vi "Boron Rod.vi"() -> ()   [LabVIEW 2020]
uses:
  <vilib>/Utility/miscctls.llb/LVAnnotationListTypeDef.ctl
  070368b1-a1f6-40e9-b446-795936455d25.vi
  <vilib>/Analysis/3filter.llb/Savitzky-Golay Filter (DBL).vi
  global/SettingVariable.vi
  <vilib>/Analysis/NI_AAL_SigProc.lvlib
  <vilib>/Analysis/NI_AALPro.lvlib
  <vilib>/Analysis/NI_AALBase.lvlib
panel:
  out "历史波形图":cluster{dbl, dbl, dbl[][]}(graph)
  in  "width":i32=60
  in  "选择反应性：":enum16{""}(ring)
  out "左选标时刻":timestamp caption="左选标时刻：" format="%<%.2X %x>T"
  out "数据点数":i32 caption="选中的数据点数："
  in  "拟合直线":bool
  out "采样间隔":dbl
  out "开始时间":timestamp
  in  "在线数据":bool
  in  "打开文件":bool
  out "反应性记录表":string[][](table) caption="计算结果记录表"
  in  "保存表格":bool
  in  "添加记录":bool
  out "提示信息":string="打开文件后，拖动波形图中的游标选取数据进行计算。"
  out "文件信息":string
  # "坐标轴与图例"
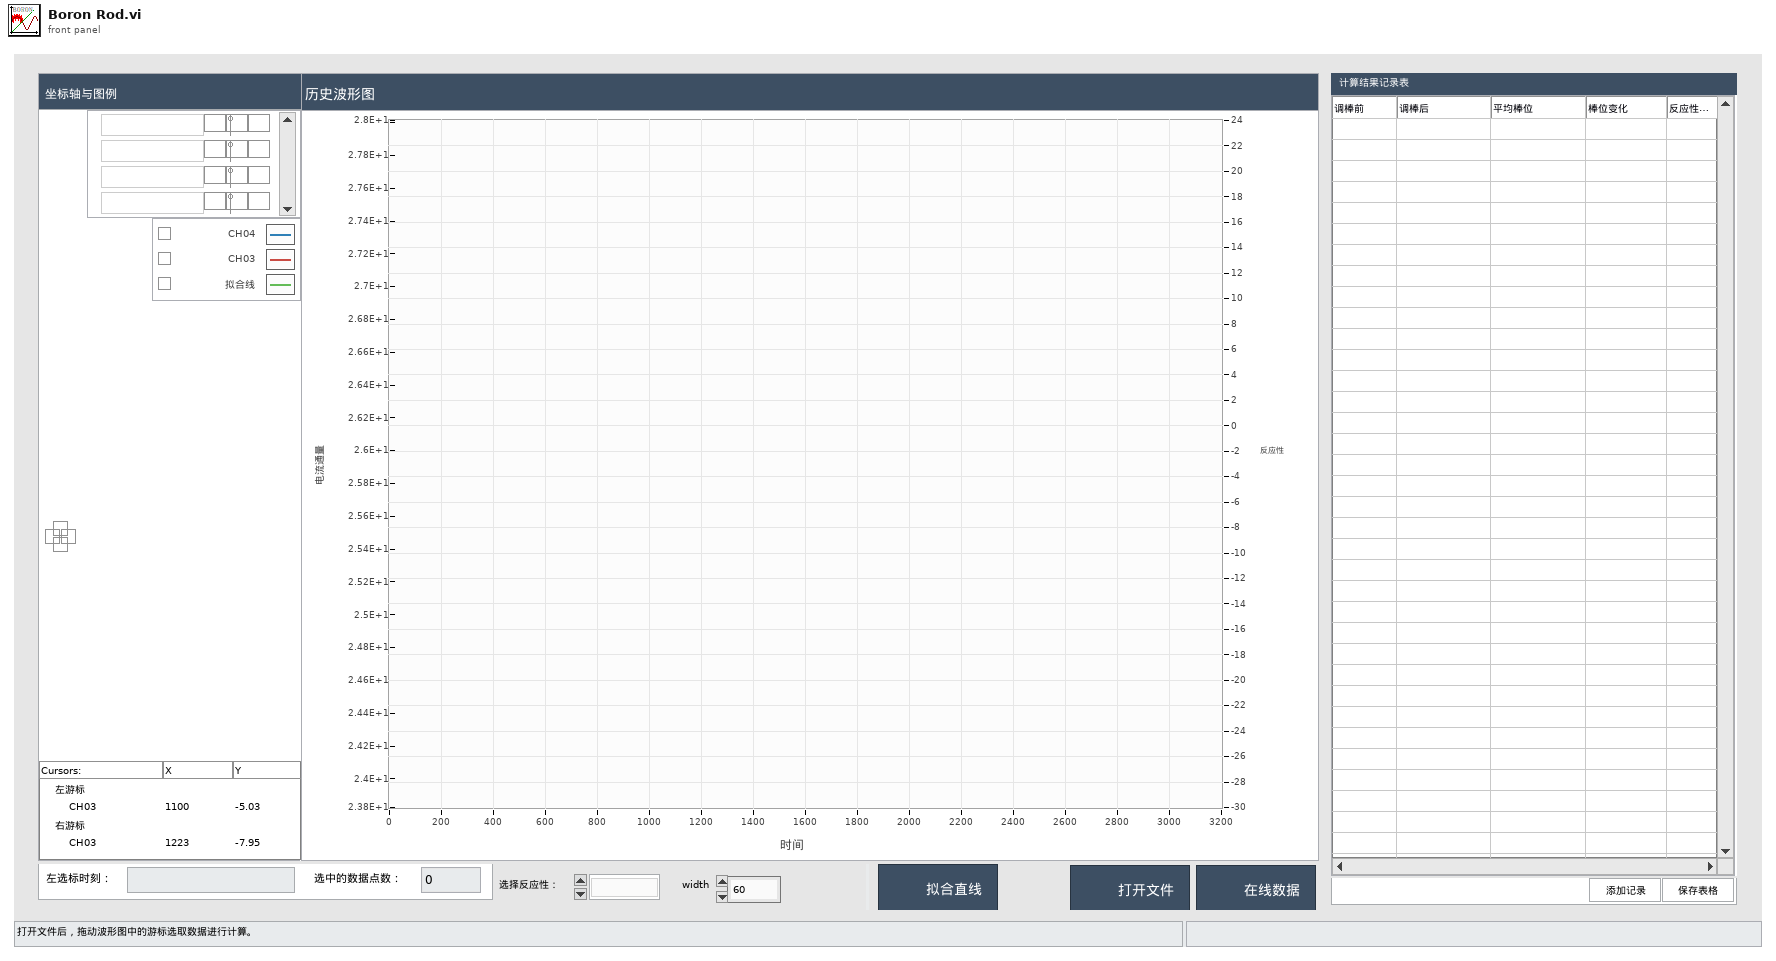
[diagram p1: front panel]
types:
  T1 = typedef "LVAnnotationListTypeDef.ctl" = cluster{"Name":string, "Color":u32, "Style":u8, "Point Style":u8, "Name Visible":bool, "Allow Drag":bool, "Annotation Mode":u32, "Plot":i32, "Index":i32, "Position":cluster{"X":dbl, "Y":dbl}, "X Scale":u32, "Y Scale":u32, "Show Arrow":bool, "Lock Name":bool, "Plot Area":i32, "Label Offset":cluster{"X":dbl, "Y":dbl}}[]
  T2 = cluster{"Name":string, "Color":u32, "Style":u8, "Point Style":u8, "Name Visible":bool, "Allow Drag":bool, "Annotation Mode":u32, "Plot":i32, "Index":i32, "Position":cluster{"X":dbl, "Y":dbl}, "X Scale":u32, "Y Scale":u32, "Show Arrow":bool, "Lock Name":bool, "Plot Area":i32, "Label Offset":cluster{"X":dbl, "Y":dbl}}
  T3 = enum16{"open", "replace", "create", "open or create", "replace or create", "replace or create with confirmation"}
  T4 = typedef "LVCursorListTypeDef.ctl" = cluster{"Name":string, "Color":u32, "Style":u8, "Point Style":u8, "Name Visible":bool, "Allow Drag":bool, "Cursor Mode":u32, "Plot":i32, "Index":i32, "Position":cluster{"X":dbl, "Y":dbl}, "X Scale":u32, "Y Scale":u32, "Watch Plots":i32[], "Watch All Plots":bool, "Plot Area":i32, "Label Offset":cluster{"X":dbl, "Y":dbl}}[]
  T5 = cluster{"Name":string, "Color":u32, "Style":u8, "Point Style":u8, "Name Visible":bool, "Allow Drag":bool, "Cursor Mode":u32, "Plot":i32, "Index":i32, "Position":cluster{"X":dbl, "Y":dbl}, "X Scale":u32, "Y Scale":u32, "Watch Plots":i32[], "Watch All Plots":bool, "Plot Area":i32, "Label Offset":cluster{"X":dbl, "Y":dbl}}
  T6 = enum32{"invalid app kind", "Development System", "Run Time System", "Student Edition", "Embedded LabVIEW", "Evaluation", "Custom"}
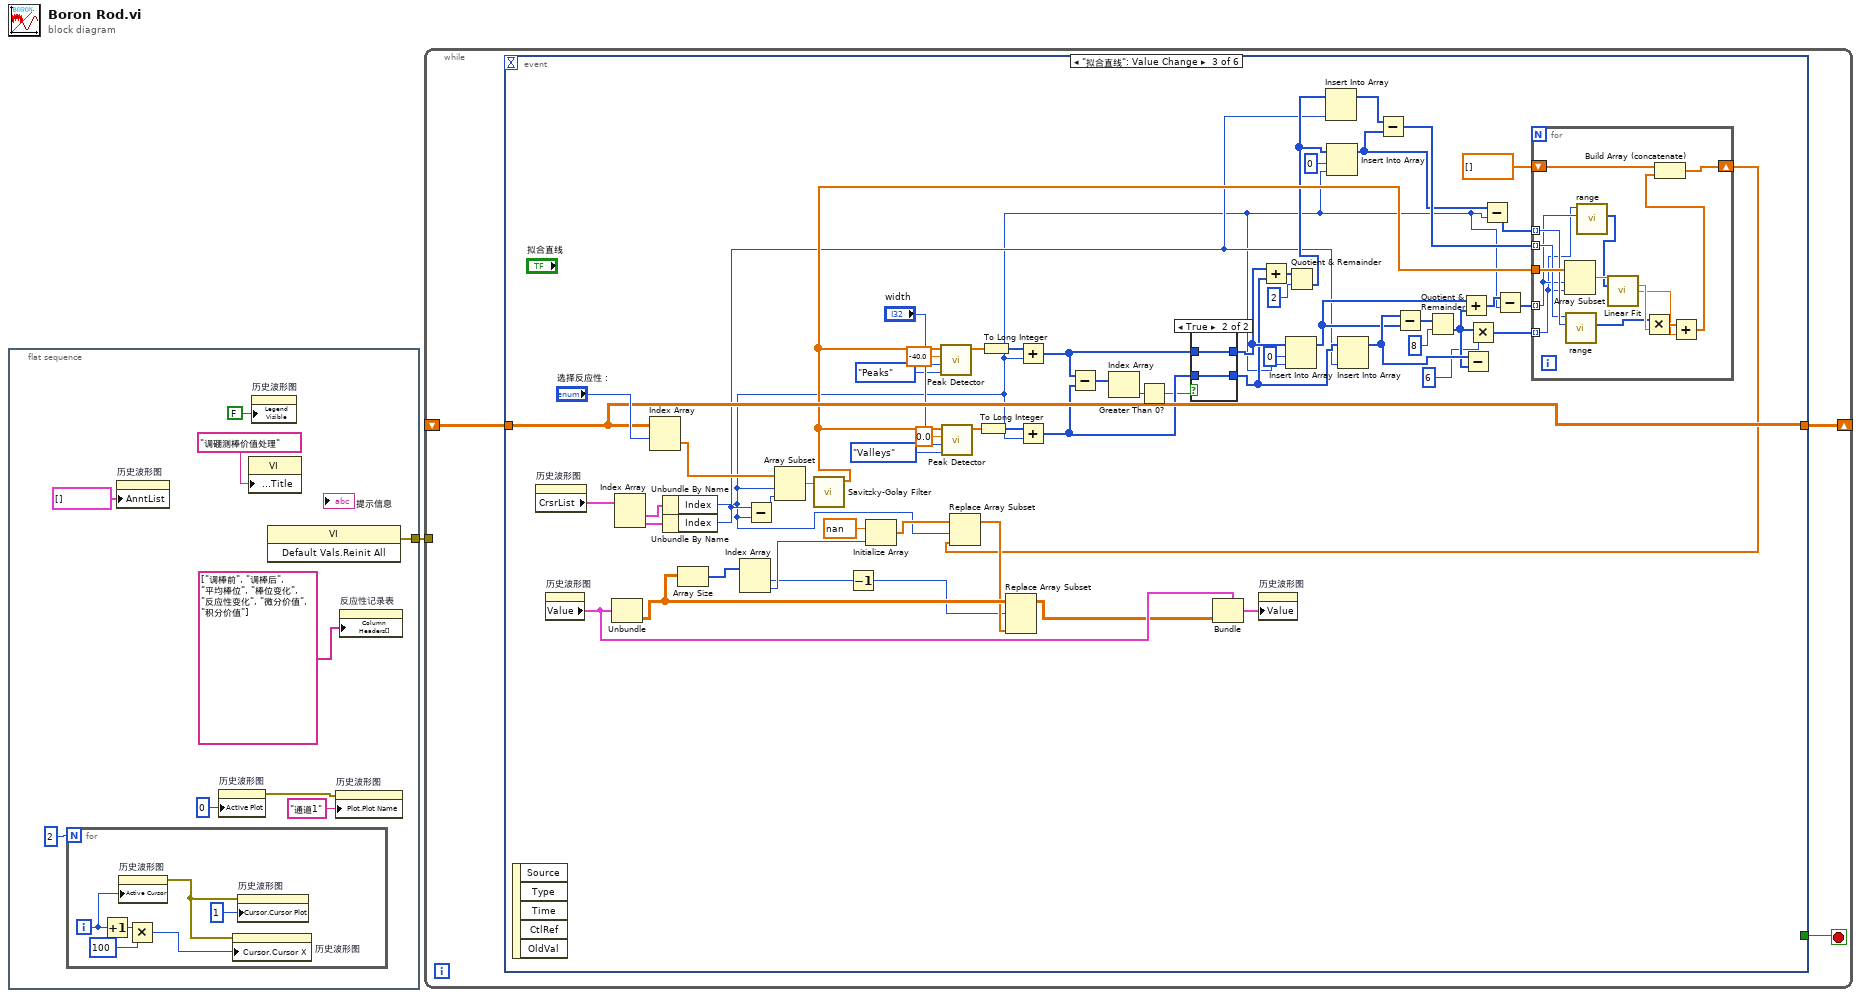
[diagram p0: block diagram]
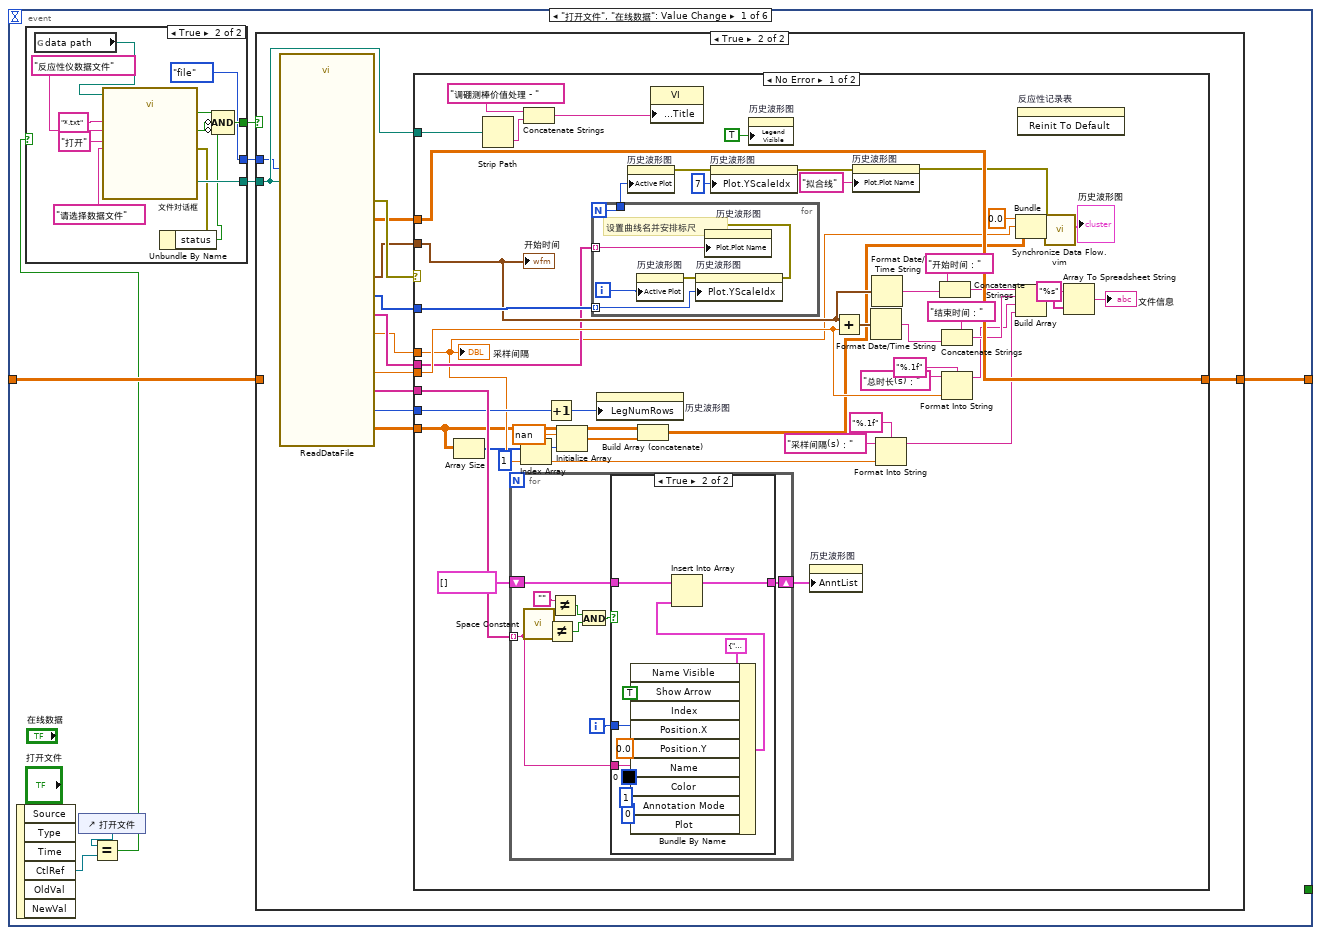
[diagram p2: hidden frame]
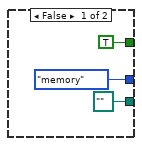
[diagram p3: hidden frame]
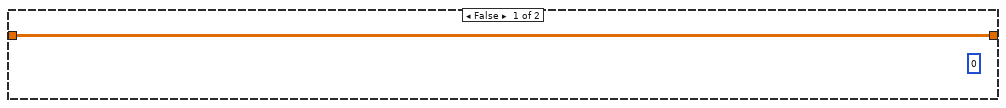
[diagram p4: hidden frame]
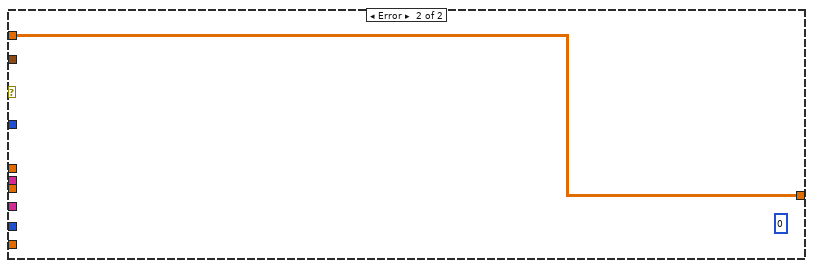
[diagram p6: hidden frame]
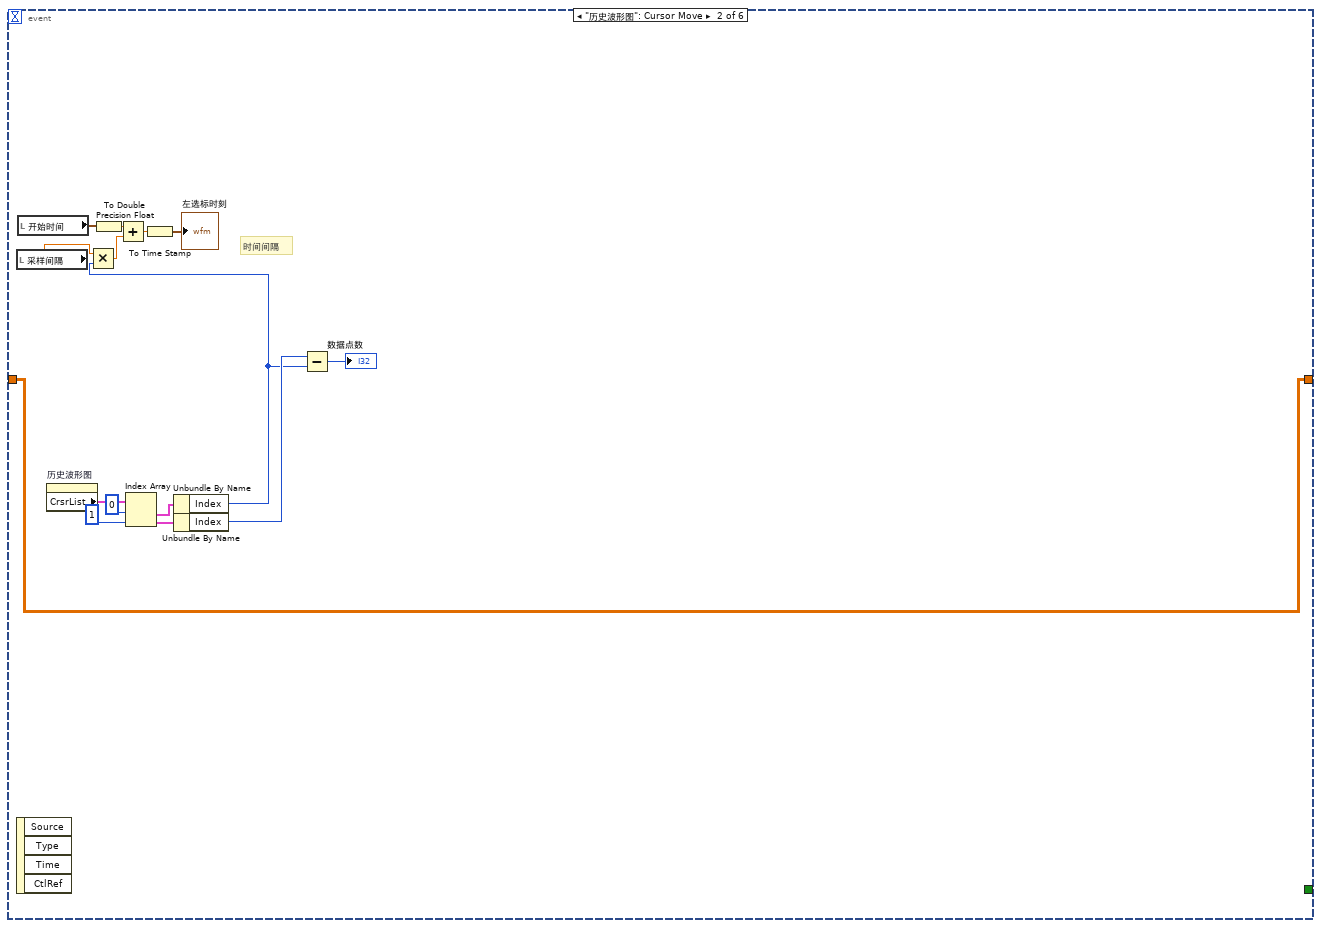
[diagram p7: hidden frame]
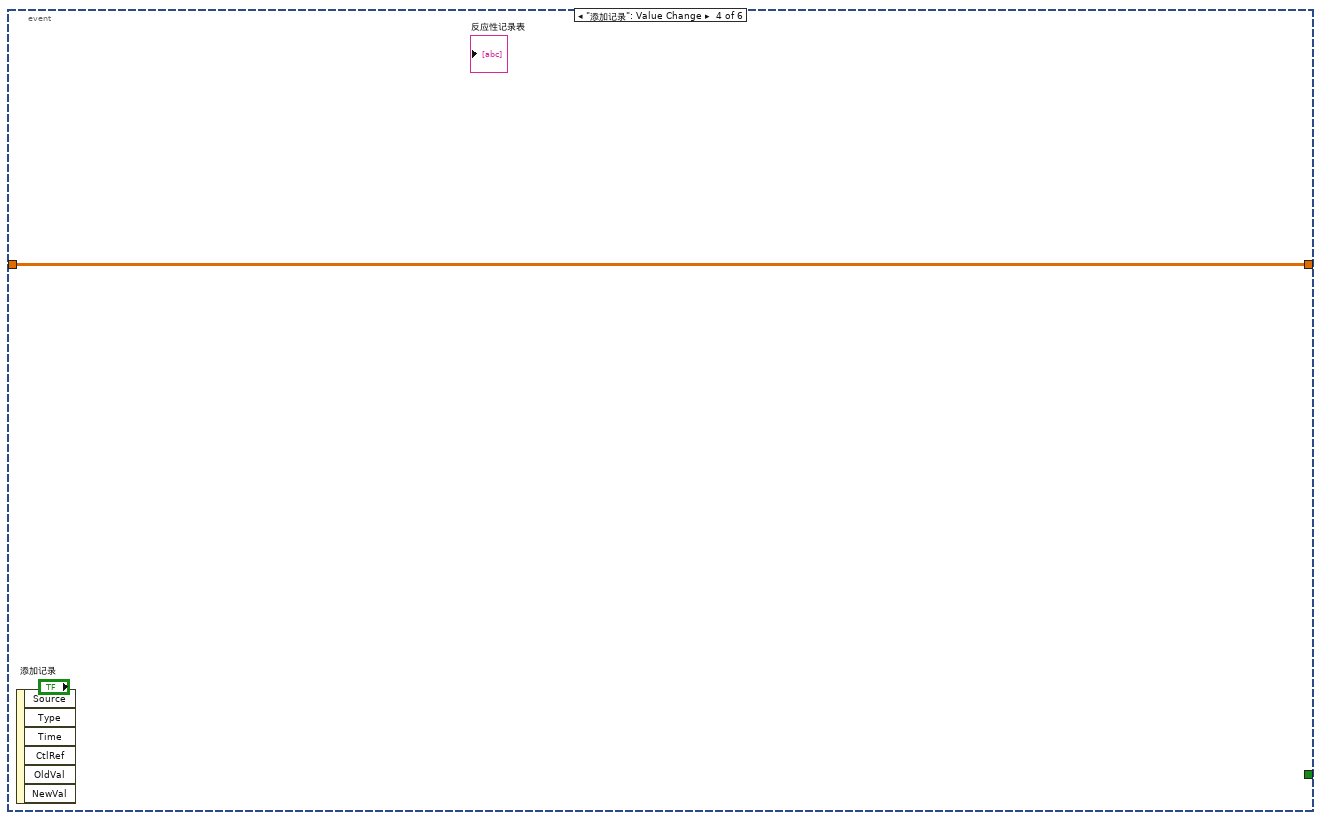
[diagram p9: hidden frame]
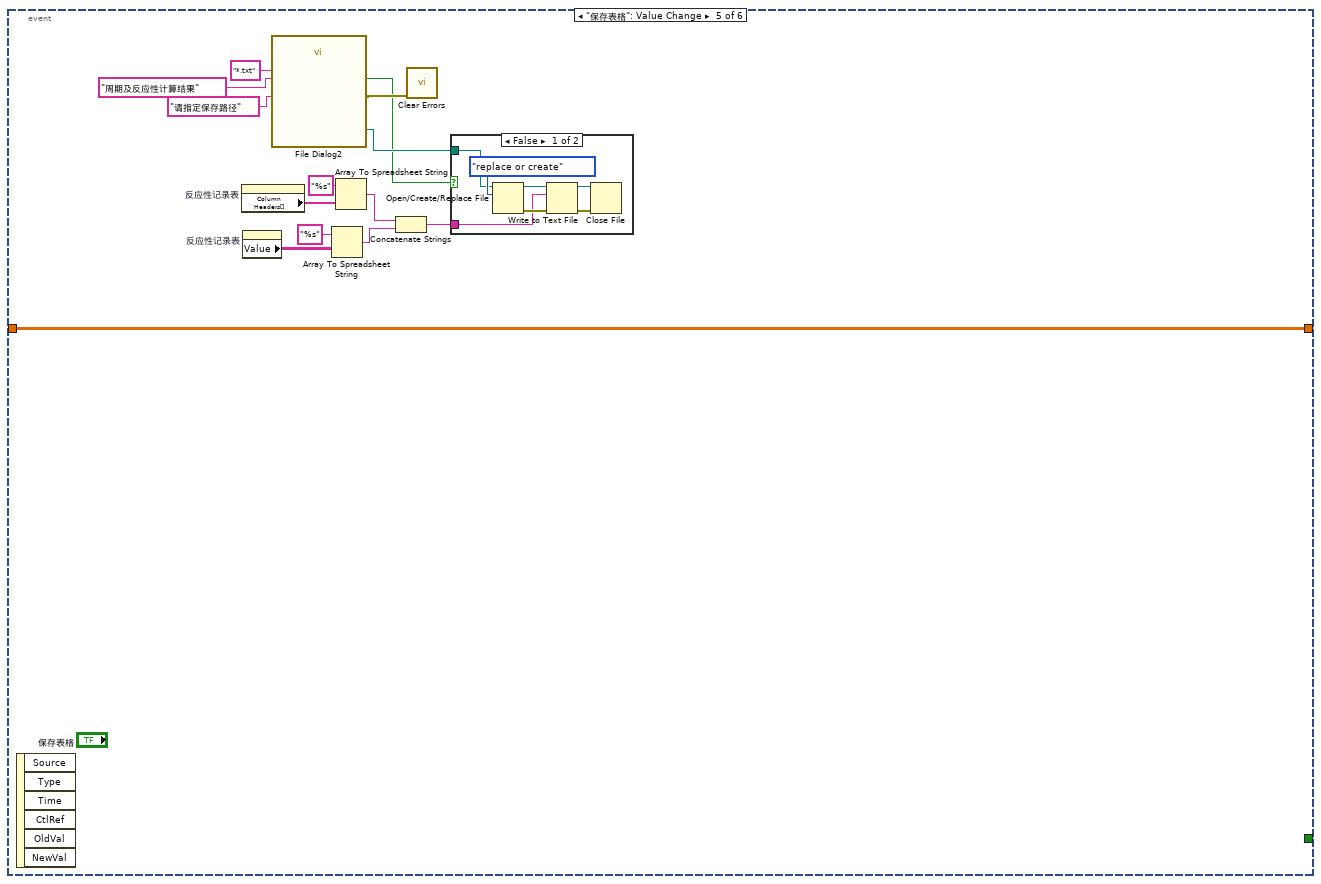
[diagram p10: hidden frame]
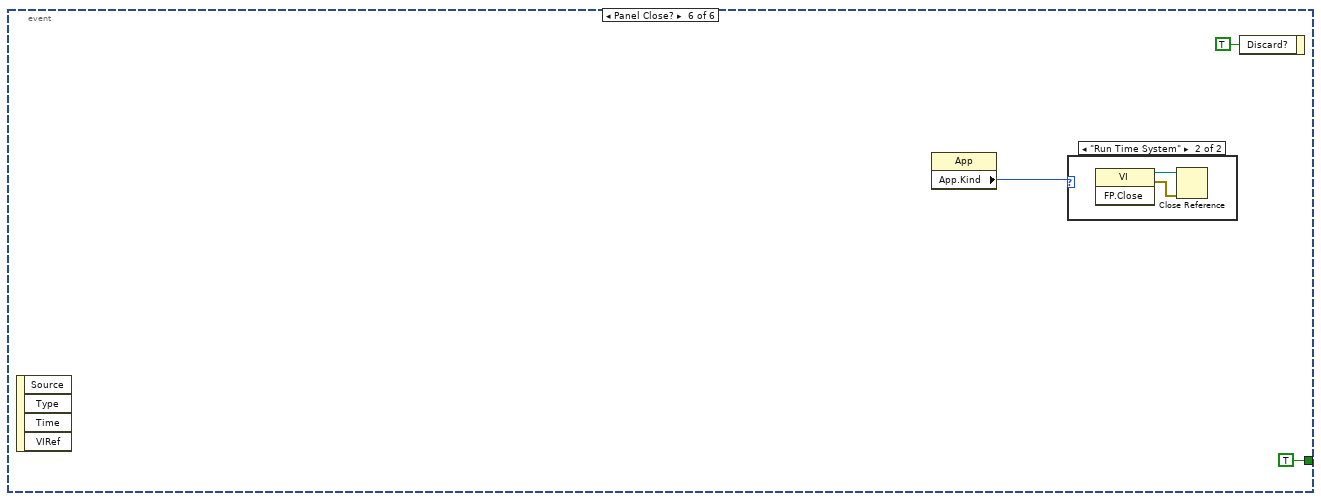
[diagram p12: hidden frame]
diagram:
  n1 = flat-sequence {
    tunnel: [w6] -> w1
    frame #0 {
      n2 = for {
        N: 2 -> [_]
        i -> [w15]
        n3 = Increment(x=w15) -> (x+1=w14:i32)
        n4 = property on="历史波形图" class="WFGraph (strict)"("Active Cursor"=w15) -> (error out=w11:errorcluster)  [unwired: 2 in, 1 out]
        n5 = Multiply(x=w14, y=100) -> (x*y=w12:i32)
        n6 = property on="历史波形图" class="WFGraph (strict)"(error in=w11, "Cursor.Cursor X"=w12) -> ()  [unwired: 1 in, 2 out]
        n7 = property on="历史波形图" class="WFGraph (strict)"(error in=w11, "Cursor.Cursor Plot"=1 ("Cursor.Cursor Index")) -> ()  [unwired: 1 in, 2 out]
      }
      n8 = property on="历史波形图" class="WFGraph (strict)"("AnntList"=T1 [] ("Annotation List")) -> ()  [unwired: 2 in, 2 out]
      n9 = property on="历史波形图" class="WFGraph (strict)"("Active Plot"=u32 0) -> (error out=w8:errorcluster)  [unwired: 2 in, 1 out]
      n10 = property class="VI"("Front Panel.Title"="调硼测棒价值处理" ("Front Panel Window:Title")) -> ()  [unwired: 2 in, 2 out]
      n11 = property on="历史波形图" class="WFGraph (strict)"("Legend Visible"=FALSE ("Legend:Visible")) -> ()  [unwired: 2 in, 2 out]
      n12 = invoke class="VI" method="Default Vals.Reinit All"() -> (error out=w6:errorcluster)  [unwired: 3 in, 2 out]
      n13 = property on="历史波形图" class="WFGraph (strict)"(error in=w8, "Plot.Plot Name"="通道1") -> ()  [unwired: 1 in, 2 out]
      n14 = property on="反应性记录表" class="Tbl (strict)"("Column Headers[]"=string[] ["调棒前", "调棒后", "平均棒位", "棒位变化", "反应性变化", "微分价值", "积分价值"] ("行首字符串[]")) -> ()  [unwired: 2 in, 2 out]
    }
  }
  n15 = while {
    shift-right: [w19] -> _
    shift-left: _ -> [w18]
    tunnel: w1 -> [_]
    stop <- w17 stop-if-true
    n16 = event shown="[2] \"拟合直线\": Value Change" {
      selector: _ -> [_ _ _ _ _ _]
      dyn-events: _ -> [_ _ _ _ _ _]
      timeout: _ -> [_ _ _ _ _ _]
      tunnel: [w26 w137 w190 w224 w238 _] -> w19
      tunnel: w18 -> [w25 w137 w190 w224 w238 _]
      tunnel: [_ _ _ _ _ TRUE] -> w17
      event "打开文件", "在线数据": Value Change {
        n17 = event-data() -> ("CtlRef"=w23:refnum<vi>)  [unwired: 1 in, 5 out]
        n18 = control-ref of="打开文件"() -> (w22:refnum<vi>)
        n19 = Equal?(x=w22, y=w23) -> (x = y?=w21:bool)
        n20 = case shown="True" w21 {
          tunnel: [path "" ("selected path") w42] -> w27
          tunnel: [TRUE w33] -> w24
          tunnel: [enum16{"file", "memory"}."memory" ("source") enum16{"file", "memory"}."file" ("source")] -> w20
          frame False {
          }
          frame True {
            n21 = global read "SettingVariable.vi" "data path"() -> (w32:path)
            n22 = call "文件对话框"("start path"=w32, "prompt"="请选择数据文件", "button label"="打开", "pattern (all files)"="*.txt", "pattern label"="反应性仪数据文件") -> ("selected path"=w42:path, "exists"=w36:bool, "cancelled"=w35:bool, "error out"=w37:errorcluster)  [unwired: 7 in]
            n23 = Unbundle By Name(w37) -> ("status"=w34:bool)
            n24 = Compound Arithmetic op=AND(w36, invert w35, invert w34) -> (w33:bool)
          }
        }
        n25 = case shown="True" w24 {
          tunnel: w27 -> [_ w46]
          tunnel: [w43 w48] -> w26
          tunnel: w25 -> [w43 _]
          tunnel: w20 -> [_ w45]
          frame False {
            (unwired) 0 ("曲线数")
          }
          frame True {
            n26 = call "ReadDataFile.vi"("file path"=w46, "source"=w45) -> ("曲线对应标尺编号"=w52:i32[], "全部数据"=w44:dbl[][], "曲线名"=w51:string[], "时间间隔"=w50:dbl, "曲线数"=w54:i32, "开始时间"=w47:timestamp, "反应性数据"=w49:dbl[][], "总时长(s)"=w55:dbl, "error out"=w56:errorcluster, "备注数组"=w53:string[])  [unwired: 1 in, 3 out]
            n27 = case shown="No Error" w56 {
              tunnel: w55 -> [w93 _]
              tunnel: w54 -> [w75 _]
              tunnel: w53 -> [w102 _]
              tunnel: w52 -> [w101 _]
              tunnel: w51 -> [w81 _]
              tunnel: w50 -> [w67 _]
              tunnel: w49 -> [w100 w132]
              tunnel: [w100 w132] -> w48
              tunnel: w47 -> [w98 _]
              tunnel: w46 -> [w77 _]
              tunnel: w44 -> [w63 _]
              frame No Error {
                n28 = Array Size(array=w63) -> (size(s)=w65:i32[])
                n29 = Strip Path(path=w77) -> (name=w78:string)  [unwired: 1 out]
                n30 = for {
                  tunnel: w102 -> [w114] mode=indexing
                  shift-right: [w116] -> w104
                  shift-left: T1 [] ("注释列表") -> [w117]
                  i -> [w118]
                  n31 = call <vilib>:"Space Constant.vi"() -> ("String"=w119:string)
                  n32 = Not Equal?(x=w119, y=w114) -> (x != y?=w112:bool)
                  n33 = Not Equal?(x="", y=w114) -> (x != y?=w113:bool)
                  n34 = And(x=w113, y=w112) -> (x .and. y?=w111:bool)
                  n35 = case shown="True" w111 {
                    tunnel: w114 -> [_ w126]
                    tunnel: w118 -> [_ w128]
                    tunnel: w117 -> [w120 w131]
                    tunnel: [w120 w130] -> w116
                    frame False {
                    }
                    frame True {
                      w129 = TRUE ("Show Arrow")
                      n36 = Bundle By Name(cluster=T2 {"Name"="", "Color"=0, "Style"=0, "Point Style"=0, "Name Visible"=FALSE, "Allow Drag"=FALSE, "Annotation Mode"=0, "Plot"=0, "Index"=0, "Position"={"X"=0.0, "Y"=0.0}, "X Scale"=0, "Y Scale"=0, "Show Arrow"=FALSE, "Lock Name"=FALSE, "Plot Area"=0, "Label Offset"={"X"=0.0, "Y"=0.0}} ("元素"), "Name Visible"=w129, "Show Arrow"=w129, "Index"=w128, "Position.X"=w128, "Position.Y"=0.0 ("Y"), "Name"=w126, "Color"=u32 0, "Annotation Mode"=u32 1, "Plot"=0) -> (w127:T2)
                      n37 = Insert Into Array(array=w131, new element=w127) -> (w130:T1)  [unwired: 1 in]
                    }
                  }
                }
                n38 = Index Array(array=w65, index=1) -> (element=w62:i32)
                n39 = Concatenate Strings("调硼测棒价值处理 - " ("string"), w78) -> (w79:string)
                n40 = Increment(x=w75) -> (x+1=w57:i32)
                n41 = Initialize Array(nan, w62) -> (w60:dbl[])
                n42 = for {
                  N -> [w105]
                  tunnel: w101 -> [w108] mode=indexing
                  tunnel: w81 -> [w106] mode=indexing
                  tunnel: [w105] -> w70
                  i -> [w107]
                  # "设置曲线名并安排标尺"
                  n43 = property on="历史波形图" class="WFGraph (strict)"("Active Plot"=w107) -> (error out=w110:errorcluster)  [unwired: 2 in, 1 out]
                  n44 = property on="历史波形图" class="WFGraph (strict)"(error in=w110, "Plot.YScaleIdx"=w108) -> (error out=w109:errorcluster)  [unwired: 1 in, 1 out]
                  n45 = property on="历史波形图" class="WFGraph (strict)"(error in=w109, "Plot.Plot Name"=w106) -> ()  [unwired: 1 in, 2 out]
                }
                n46 = property on="历史波形图" class="WFGraph (strict)"("LegNumRows"=w57) -> ()  [unwired: 2 in, 2 out]
                n47 = property on="历史波形图" class="WFGraph (strict)"("Active Plot"=w70) -> (error out=w72:errorcluster)  [unwired: 2 in, 1 out]
                n48 = Build Array (concatenate)(w63, w60) -> (w66:dbl[][])
                n49 = property class="VI"("Front Panel.Title"=w79) -> ()  [unwired: 2 in, 2 out]
                n50 = property on="历史波形图" class="WFGraph (strict)"(error in=w72, "Plot.YScaleIdx"=u32 7 ("Plot.Y Scale Index")) -> (error out=w73:errorcluster)  [unwired: 1 in, 1 out]
                n51 = property on="历史波形图" class="WFGraph (strict)"("Legend Visible"=TRUE ("Legend:Visible")) -> ()  [unwired: 2 in, 2 out]
                n52 = property on="历史波形图" class="WFGraph (strict)"("AnntList"=w104) -> ()  [unwired: 2 in, 2 out]
                n53 = Add(x=w98, y=w93) -> (x+y=w99:timestamp)
                n54 = property on="历史波形图" class="WFGraph (strict)"(error in=w73, "Plot.Plot Name"="拟合线") -> (error out=w58:errorcluster)  [unwired: 1 in, 1 out]
                n55 = Format Date/Time String(seconds (now)=w99) -> (date/time string=w94:string)  [unwired: 2 in]
                n56 = Format Date/Time String(seconds (now)=w98) -> (date/time string=w96:string)  [unwired: 2 in]
                n57 = Format Into String(format string="%.1f", initial string="采样间隔(s)：", w67) -> (resulting string=w85:string)  [unwired: 1 in, 1 out]
                n58 = Concatenate Strings("开始时间：" ("string"), w96) -> (w90:string)
                n59 = Concatenate Strings("结束时间：" ("string"), w94) -> (w87:string)
                n60 = Format Into String(format string="%.1f", initial string="总时长(s)：", w93) -> (resulting string=w86:string)  [unwired: 1 in, 1 out]
                n61 = Bundle(0.0, "时间间隔"=w67, w66) -> (w69:cluster{dbl, "时间间隔":dbl, dbl[][]})  [unwired: 1 in]
                n62 = Build Array(w90, w87, w86, w85) -> (w89:string[])
                n63 = invoke on="反应性记录表" class="Tbl (strict)" method="Reinit To Default"() -> ()  [unwired: 3 in, 3 out]
                n64 = call "Synchronize Data Flow.vim"("input 2"=w69, "input 1"=w58) -> ("output 2"=→"历史波形图":cluster{dbl, "时间间隔":dbl, dbl[][]})  [unwired: 2 in, 3 out]
                n65 = Array To Spreadsheet String(array=w89, 3:"%s" ("format string")) -> (spreadsheet string=→"文件信息":string)  [unwired: 1 in]
                "开始时间" <- w98
                "采样间隔" <- w67
              }
              frame Error {
                (unwired) 0 ("曲线数")
              }
            }
          }
        }
      }
      event "历史波形图": Cursor Move {
        # "时间间隔"
        n66 = local read "采样间隔"() -> (w135:dbl)
        n67 = event-data() -> ()  [unwired: 1 in, 4 out]
        n68 = local read "开始时间"() -> (w136:timestamp)
        n69 = property on="历史波形图" class="WFGraph (strict)"() -> ("CrsrList"=w143:T4)  [unwired: 2 in, 2 out]
        n70 = To Double Precision Float(number=w136) -> (double precision float=w142:dbl)
        n71 = Index Array(array=w143, index #1=0 ("index"), index #2=1 ("index")) -> (element #1=w145:T5, element #2=w147:T5)
        n72 = Unbundle By Name(w145) -> ("Index"=w133:i32)
        n73 = Multiply(x=w135, y=w133) -> (x*y=w139:dbl)
        n74 = Add(x=w142, y=w139) -> (x+y=w141:dbl)
        n75 = To Time Stamp(1:w141) -> (0:→"左选标时刻":timestamp)
        n76 = Unbundle By Name(w147) -> ("Index"=w138:i32)
        n77 = Subtract(x=w138, y=w133) -> (x-y=→"数据点数":i32)
      }
      event "拟合直线": Value Change {
        n78 = event-data() -> ()  [unwired: 1 in, 5 out]
        n79 = property on="历史波形图" class="WFGraph (strict)"() -> ("CrsrList"=w203:T4)  [unwired: 2 in, 2 out]
        n80 = property on="历史波形图" class="WFGraph (strict)"() -> ("Value"=w193:cluster{dbl, dbl, dbl[][]})  [unwired: 2 in, 2 out]
        n81 = Unbundle(w193) -> (w199:dbl[][])  [unwired: 2 out]
        n82 = Index Array(array=w203) -> (element #1=w204:T5, element #2=w205:T5)  [unwired: 2 in]
        n83 = Index Array(array=w190, index (row)="选择反应性：") -> (element=w201:dbl[])  [unwired: 1 in]
        n84 = Unbundle By Name(w204) -> ("Index"=w149:i32)
        n85 = Unbundle By Name(w205) -> ("Index"=w155:i32)
        n86 = Array Size(array=w199) -> (size(s)=w198:i32[])
        n87 = Index Array(array=w198) -> (element #1=w194:i32, element #2=w197:i32)  [unwired: 2 in]
        n88 = Subtract(x=w155, y=w149) -> (x-y=w200:i32)
        n89 = Array Subset(array=w201, index=w149, length=w200) -> (w163:dbl[])
        n90 = call-poly <vilib>:"Savitzky-Golay Filter.vi"("X"=w163) -> ("Filtered X"=w162:dbl[])  [unwired: 9 in, 1 out]
        n91 = Decrement(x=w194) -> (x-1=w189:i32)
        n92 = Initialize Array(nan ("element"), w197) -> (w188:dbl[])
        n93 = call <vilib>:"Peak Detector.vi"("peaks/valleys"=enum32{"Peaks", "Valleys"}."Peaks", "width"="width", "threshold"=-40.0, "X"=w162) -> ("Locations"=w187:dbl[])  [unwired: 3 in, 4 out]
        n94 = call <vilib>:"Peak Detector.vi"("peaks/valleys"=enum32{"Peaks", "Valleys"}."Valleys", "width"="width", "threshold"=0.0, "X"=w162) -> ("Locations"=w183:dbl[])  [unwired: 3 in, 4 out]
        n95 = To Long Integer(number=w183) -> (32bit integer=w179:i32[])
        n96 = To Long Integer(number=w187) -> (32bit integer=w180:i32[])
        n97 = Add(x=w180, y=w149) -> (x+y=w168:i32[])
        n98 = Add(x=w179, y=w149) -> (x+y=w167:i32[])
        n99 = Subtract(x=w168, y=w167) -> (x-y=w181:i32[])
        n100 = Index Array(array=w181) -> (element=w182:i32)  [unwired: 1 in]
        n101 = Greater Than 0?(x=w182) -> (x > 0?=w166:bool)
        n102 = case shown="True" w166 {
          tunnel: [w206 w209] -> w161
          tunnel: w168 -> [w207 w209]
          tunnel: [w207 w208] -> w160
          tunnel: w167 -> [w206 w208]
          frame False {
          }
          frame True {
          }
        }
        n103 = Add(x=w161, y=w160) -> (x+y=w159:i32[])
        n104 = Insert Into Array(array=w161, index=0, new element=w149) -> (w172:i32[])
        n105 = Quotient & Remainder(x=w159, y=2) -> (floor(x/y)=w156:i32[])  [unwired: 1 out]
        n106 = Insert Into Array(array=w156, new element=w155) -> (w154:i32[])  [unwired: 1 in]
        n107 = Insert Into Array(array=w156, index=0, new element=w149) -> (w151:i32[])
        n108 = Insert Into Array(array=w160, new element=w155) -> (w176:i32[])  [unwired: 1 in]
        n109 = Subtract(x=w154, y=w151) -> (x-y=w153:i32[])
        n110 = Subtract(x=w176, y=w172) -> (x-y=w171:i32[])
        n111 = Quotient & Remainder(x=w171, y=8) -> (floor(x/y)=w175:i32[])  [unwired: 1 out]
        n112 = Add(x=w172, y=w175) -> (x+y=w150:i32[])
        n113 = Subtract(x=w176, y=w175) -> ()  [unwired: 1 out]
        n114 = Multiply(x=w175, y=6) -> (x*y=w173:i32[])
        n115 = Subtract(x=w151, y=w149) -> (x-y=w152:i32[])
        n116 = Subtract(x=w150, y=w149) -> (x-y=w148:i32[])
        n117 = for {
          tunnel: w162 -> [w223]
          tunnel: w148 -> [w219] mode=indexing
          tunnel: w173 -> [w218] mode=indexing
          tunnel: w152 -> [w221] mode=indexing
          tunnel: w153 -> [w220] mode=indexing
          shift-right: [w210] -> w169
          shift-left: dbl[] [] -> [w212]
          n118 = Array Subset(array=w223, index=w219, length=w218) -> (w222:dbl[])
          n119 = call "range.vi"("x0"=w221, "N"=w220) -> ("Range"=w215:i32[])  [unwired: 9 in]
          n120 = call "range.vi"("x0"=w219, "N"=w218) -> ("Range"=w217:i32[])  [unwired: 9 in]
          n121 = call <vilib>:"Linear Fit.vi"("Y"=w222, "X"=w217) -> ("slope"=w216:dbl, "intercept"=w213:dbl)  [unwired: 9 in, 3 out]
          n122 = Multiply(x=w215, y=w216) -> (x*y=w214:dbl[])
          n123 = Add(x=w214, y=w213) -> (x+y=w211:dbl[])
          n124 = Build Array (concatenate)(w212, w211) -> (w210:dbl[])
        }
        n125 = Replace Array Subset(array=w188, new element=w169, index=w149) -> (w195:dbl[])
        n126 = Replace Array Subset(array=w199, new element=w195, index (row)=w189) -> (w192:dbl[][])  [unwired: 1 in]
        n127 = Bundle(cluster=w193, w192) -> (w191:cluster{dbl, dbl, dbl[][]})  [unwired: 2 in]
        n128 = property on="历史波形图" class="WFGraph (strict)"("Value"=w191) -> ()  [unwired: 2 in, 2 out]
      }
      event "添加记录": Value Change {
        n129 = event-data() -> ()  [unwired: 1 in, 6 out]
      }
      event "保存表格": Value Change {
        n130 = event-data() -> ()  [unwired: 1 in, 6 out]
        n131 = property on="反应性记录表" class="Tbl (strict)"() -> ("Column Headers[]"=w237:string[])  [unwired: 2 in, 2 out]
        n132 = property on="反应性记录表" class="Tbl (strict)"() -> ("Value"=w234:string[][])  [unwired: 2 in, 2 out]
        n133 = call "File Dialog2"("prompt"="请指定保存路径" ("提示"), "pattern (all files)"="*.txt" ("类型（所有文件）"), "pattern label"="周期及反应性计算结果" ("默认名称")) -> ("selected path"=w231:path, "cancelled"=w230:bool, "error out"=w232:errorcluster)  [unwired: 9 in, 1 out]
        n134 = Array To Spreadsheet String(array=w234, 3:"%s" ("format string")) -> (spreadsheet string=w233:string)  [unwired: 1 in]
        n135 = Array To Spreadsheet String(array=w237, 3:"%s" ("格式字符串")) -> (spreadsheet string=w236:string)  [unwired: 1 in]
        n136 = Concatenate Strings(w236, w233) -> (w235:string)
        n137 = call <vilib>:"Clear Errors.vi"("error in (no error)"=w232) -> ()  [unwired: 5 in, 2 out]
        n138 = case shown="False" w230 {
          tunnel: w235 -> [w240 _]
          tunnel: w231 -> [w239 _]
          frame False {
            n139 = Open/Create/Replace File(file path (use dialog)=w239, operation (0:open)=T3."replace or create") -> (refnum out=w243:refnum<file>, error out=w245:errorcluster)  [unwired: 4 in, 1 out]
            n140 = Write to Text File(file (use dialog)=w243, text=w240, error in=w245) -> (refnum out=w242:refnum<file>, error out=w241:errorcluster)  [unwired: 1 in, 1 out]
            n141 = Close File(refnum=w242, error in=w241) -> ()  [unwired: 2 out]
          }
          frame True {
          }
        }
      }
      event Panel Close? {
        n142 = event-data() -> ()  [unwired: 1 in, 4 out]
        n143 = property class="App"() -> ("App.Kind"=w246:T6)  [unwired: 2 in, 2 out]
        n144 = case shown="\"Run Time System\"" w246 {
          frame "Development System", Default {
          }
          frame "Run Time System" {
            n145 = invoke class="VI" method="FP.Close"() -> (reference out=w249:refnum<vi>, error out=w250:errorcluster)  [unwired: 3 in, 1 out]
            n146 = Close Reference(reference=w249, error in (no error)=w250) -> ()  [unwired: 1 out]
          }
        }
        n147 = event-data("Discard?"=TRUE) -> ()  [unwired: 1 in, 1 out]
      }
    }
  }
